vi "Teardown.vi"(11 "Event Transport in":refnum<class "Event Transport.lvclass">) -> (2 "Unheard Msgs":refnum<class "Msg.lvclass">[](array[class]))   [LabVIEW 2020, in "jettl.lvlib" / "Event Transport.lvlib" / "Event Transport.lvclass"]
uses:
  Event Transport.lvclass
  Event Transport.lvclass/Event Transport.ctl
  Msg/Msg.lvclass
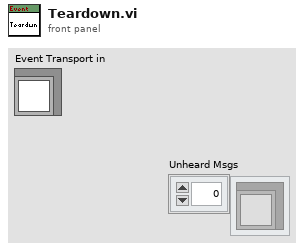
[diagram p1: front panel]
types:
  T1 = typedef "jettl.lvlib/Msg Attributes.ctl" = cluster{"Msg":refnum<class "Msg.lvclass">, "Msg Input":refnum<class "Msg Input.lvclass">, "Msg Output":refnum<class "Msg Output.lvclass">, "Teller":T2}
  T2 = typedef "jettl.lvlib/Teller.ctl" = cluster{"Absolute Time":timestamp, "Relative Time":dbl, "Alias":string, "Relation":T3}
  T3 = typedef "jettl.lvlib/Relation.ctl" = enum16{"Self", "Parent", "Child"}
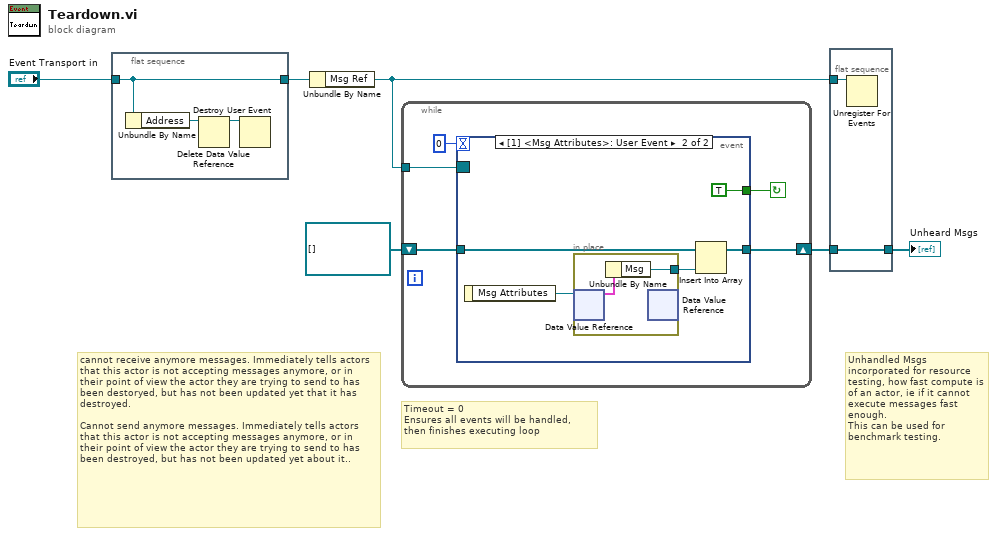
[diagram p0: block diagram]
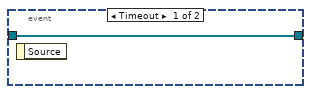
[diagram p2: hidden frame]
diagram:
  # "Unhandled Msgs incorporated for resource testing, how fast compute is of an actor, ie if it cannot execute messages fast enough.\nThis can be used for benchmark testing."
  # "Timeout = 0\nEnsures all events will be handled, then finishes executing loop"
  # "cannot receive anymore messages. Immediately tells actors that this actor is not accepting messages anymore, or in their point of view the actor they are trying to send to has been destoryed, but has not been updated yet that it has destroyed.\n\nCannot send anymore messages. Immediately tells actors that this actor is not accepting messages anymore, or in their point of view the actor they are trying to send to has been destroyed, but has not been updated yet about it.."
  n1 = flat-sequence {
    tunnel: "Event Transport in" -> [w9]
    tunnel: [w9] -> w4
    frame #0 {
      n2 = Unbundle By Name(w9) -> ("Address"=w7:refnum<data-value>)
      n3 = Delete Data Value Reference(data value reference=w7) -> (data value=w8:refnum<user-event>)  [unwired: 1 in, 1 out]
      n4 = Destroy User Event(user event=w8) -> ()  [unwired: 1 in, 1 out]
    }
  }
  n5 = Unbundle By Name(w4) -> ("Msg Ref"=w3:refnum<event-registration>)
  n6 = while {
    shift-right: [w13] -> w1
    shift-left: refnum<class "Msg.lvclass">[] [] -> [w14]
    tunnel: w3 -> [w12]
    stop <- w11 continue-if-true
    n7 = event shown="[1] <Msg Attributes>: User Event" {
      selector: w12 -> [_ _]
      dyn-events: _ -> [_ _]
      timeout: 0 -> [_ _]
      tunnel: w14 -> [w15 w20]
      tunnel: [w15 w19] -> w13
      tunnel: [_ TRUE] -> w11
      event Timeout {
        n8 = event-data() -> ()  [unwired: 1 in, 1 out]
      }
      event User Event {
        n9 = event-data() -> ("Msg Attributes"=w17:refnum<data-value>)  [unwired: 1 in]
        n10 = in-place {
          in-place-border: [w21] -> w16
          n11 = in-place-dvr #1(w17) -> (w22:T1)  [unwired: 1 out]
          n12 = Unbundle By Name(w22) -> ("Msg"=w21:refnum<class "Msg.lvclass">)
          n13 = in-place-dvr #1() -> ()  [unwired: 1 in, 2 out]
        }
        n14 = Insert Into Array(array=w20, new element=w16) -> (w19:refnum<class "Msg.lvclass">[])  [unwired: 1 in]
      }
    }
  }
  n15 = flat-sequence {
    tunnel: w3 -> [w24]
    tunnel: [w23] -> w2
    tunnel: w1 -> [w23]
    frame #0 {
      n16 = Unregister For Events(event registration refnum=w24) -> ()  [unwired: 1 in, 1 out]
    }
  }
  "Unheard Msgs" <- w2
